vi "Get Terminal Predecessors.vi"(7 "Selected":string, 8 "error in (no error)":errorcluster, 11 "Terminals[] in":refnum<vi>[](array[refnum])) -> (0 "error out":errorcluster, 3 "Terminals[] out":refnum<vi>[](array[refnum]), 5 "2nd Order Queries":string[][](array[string]))   [LabVIEW 2020]
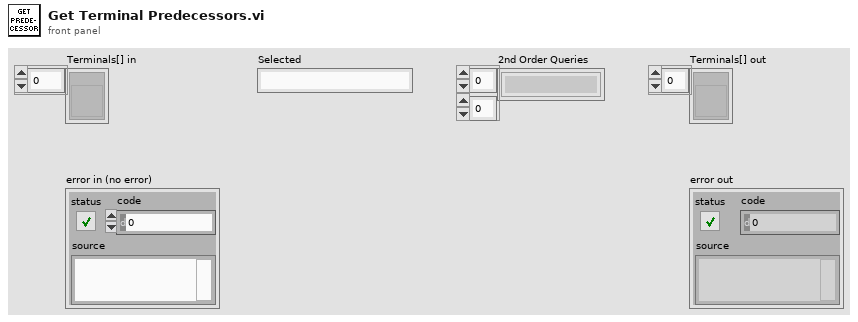
[diagram p1: front panel]
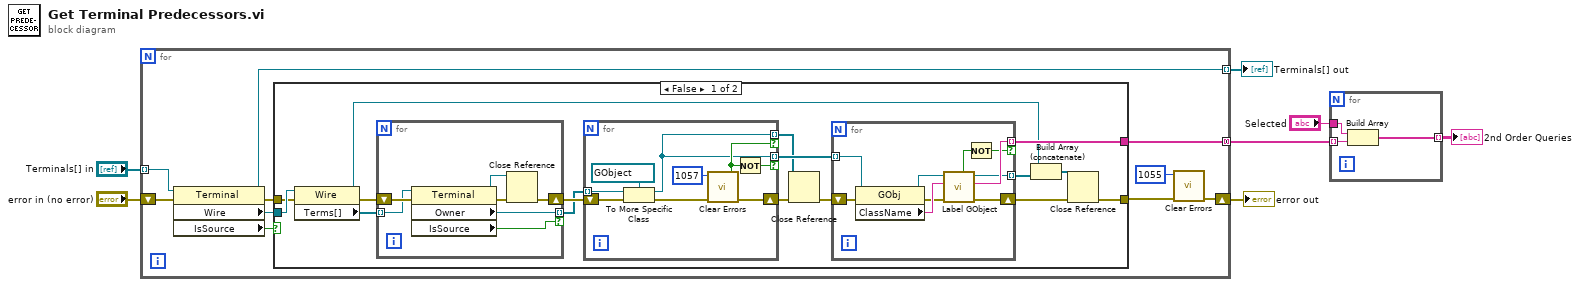
[diagram p0: block diagram]
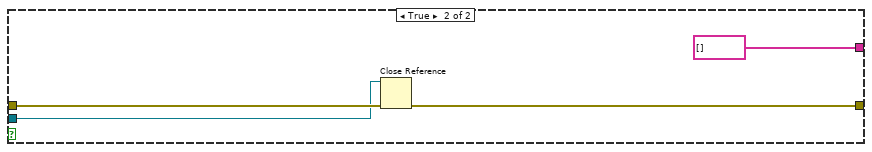
[diagram p2: hidden frame]
diagram:
  n1 = for {
    shift-right: [w8] -> w6
    shift-left: "error in (no error)" -> [w17]
    tunnel: [w15] -> w3 mode=concatenating
    tunnel: "Terminals[] in" -> [w13] mode=indexing
    tunnel: [w12] -> w4 mode=indexing
    n2 = property on="Property Node" class="Terminal"(reference=w13, error in=w17) -> (reference out=w12:refnum<vi>, error out=w16:errorcluster, "Wire"=w11:refnum<vi>, "IsSource"=w14:bool)
    n3 = case shown="False" w14 {
      tunnel: w16 -> [w28 w62]
      tunnel: [w25 w60] -> w9
      tunnel: [w30 string[] []] -> w15
      tunnel: w11 -> [w29 w61]
      frame False {
        n4 = property on="Property Node" class="Wire"(reference=w29, error in=w28) -> (reference out=w20:refnum<vi>, error out=w18:errorcluster, "Terms[]"=w27:refnum<vi>[])
        n5 = for {
          tunnel: w27 -> [w39] mode=indexing
          shift-right: [w35] -> w33
          shift-left: w18 -> [w40]
          tunnel: [w38] -> w32 mode=indexing if=w37
          n6 = property on="Property Node" class="Terminal"(reference=w39, error in=w40) -> (reference out=w34:refnum<vi>, error out=w36:errorcluster, "Owner"=w38:refnum<vi>, "IsSource"=w37:bool)
          n7 = Close Reference(reference=w34, error in (no error)=w36) -> (error out=w35:errorcluster)
        }
        n8 = for {
          shift-right: [w44] -> w24
          shift-left: w33 -> [w48]
          tunnel: w32 -> [w47] mode=indexing
          tunnel: [w41] -> w31 mode=indexing if=w43
          tunnel: [w41] -> w19 mode=indexing if=w42
          n9 = To More Specific Class(target class=refnum<vi> refnum ("reference"), reference=w47, error in=w48) -> (specific class reference=w41:refnum<vi>, error out=w45:errorcluster)
          n10 = call <vilib>:"Clear Errors.vi"("error in (no error)"=w45, "specific error code to clear (0: all)"=1057) -> ("error out"=w44:errorcluster, "specific error cleared?"=w42:bool)  [unwired: 4 in]
          n11 = Not(x=w42) -> (.not. x?=w43:bool)
        }
        n12 = Close Reference(reference=w19, error in (no error)=w24) -> (error out=w23:errorcluster)
        n13 = for {
          shift-right: [w55] -> w26
          shift-left: w23 -> [w56]
          tunnel: [w54] -> w30 mode=indexing if=w51
          tunnel: w31 -> [w53] mode=indexing
          tunnel: [w50] -> w21 mode=indexing
          n14 = property class="GObj"(reference=w53, error in=w56) -> (reference out=w57:refnum<vi>, error out=w58:errorcluster, "ClassName"=w59:string)
          n15 = call "Label GObject.vi"("error in"=w58, "GObject ClassName"=w59, "GObject Reference In"=w57) -> ("error out"=w55:errorcluster, "Label"=w54:string, "GObject Reference out"=w50:refnum<vi>, "Excluded?"=w52:bool)  [unwired: 4 in, 1 out]
          n16 = Not(x=w52) -> (.not. x?=w51:bool)
        }
        n17 = Build Array (concatenate)(w20, w21) -> (w22:refnum<vi>[])
        n18 = Close Reference(reference=w22, error in (no error)=w26) -> (error out=w25:errorcluster)
      }
      frame True {
        n19 = Close Reference(reference=w61, error in (no error)=w62) -> (error out=w60:errorcluster)
      }
    }
    n20 = call <vilib>:"Clear Errors.vi"("error in (no error)"=w9, "specific error code to clear (0: all)"=1055) -> ("error out"=w8:errorcluster)  [unwired: 4 in, 1 out]
  }
  "error out" <- w6
  "Terminals[] out" <- w4
  n21 = for {
    tunnel: w3 -> [w66] mode=indexing
    tunnel: "Selected" -> [w65]
    tunnel: [w64] -> w1 mode=indexing
    n22 = Build Array(w65, w66) -> (w64:string[])
  }
  "2nd Order Queries" <- w1
